vi "Read B.vi"(8 "error in (no error)":errorcluster, 11 "Quadratic in":refnum<class "Quadratic.lvclass">) -> (0 "error out":errorcluster, 2 "B":dbl, 3 "Quadratic out":refnum<class "Quadratic.lvclass">)   [LabVIEW 2020, in "Data Generators.lvlib" / "Quadratic.lvclass"]
uses:
  Quadratic.lvclass
  Quadratic.lvclass/Quadratic.ctl
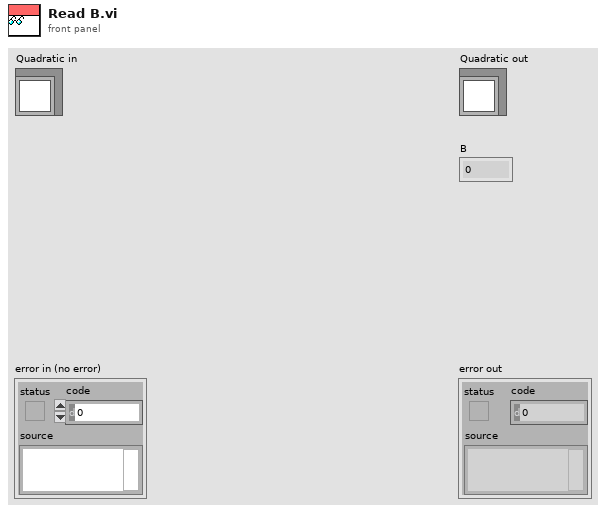
[diagram p1: front panel]
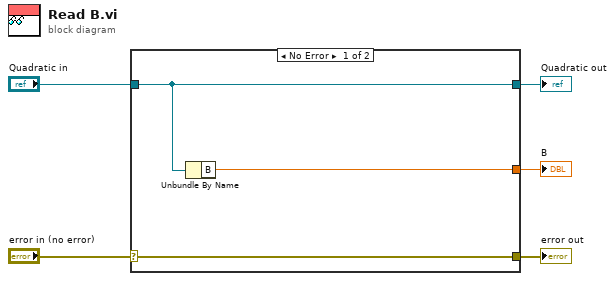
[diagram p0: block diagram]
diagram:
  n1 = case shown="No Error" "error in (no error)" {
    selector: "error in (no error)" -> [w8 w9]
    tunnel: [w8 w9] -> w4
    tunnel: [w7 w10] -> w2
    tunnel: "Quadratic in" -> [w7 w10]
    tunnel: [w6 _] -> w1
    frame No Error {
      n2 = Unbundle By Name(w7) -> ("B"=w6:dbl)
    }
    frame Error {
    }
  }
  "error out" <- w4
  "Quadratic out" <- w2
  "B" <- w1
